vi "Define.vi"(11 "Collection Definition":T1) -> (3 "Entity Collection out":refnum<class "Entity Collection.lvclass">)   [LabVIEW 2020, in "Conditu2.lvlib" / "Columns.lvlib" / "Entity Collection.lvclass"]
uses:
  Entity Collection.lvclass
  C:/dev/lv20CE/lv-conditum-tools/Conditum-Clone/Columns/Relation/Relation.lvclass
  Collection Definition.ctl
  Relation/Relation Info.ctl
  Relation Mapping.ctl
  Relation/Relation Definition.ctl
  Type/Definition.ctl
  Type/Type.lvclass/Type.ctl
  Relation/Relation.lvclass/Relation.ctl
  Type/Define Type.vi
  Relation/Relation.lvclass
  C:/dev/lv20CE/lv-conditum-tools/Conditum-Clone/Columns/Type/Type.lvclass
  Type/Type.lvclass
  Conditu2.lvlib
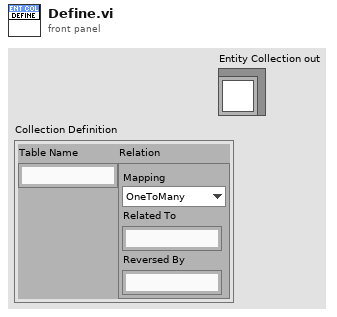
[diagram p1: front panel]
types:
  T1 = typedef "Conditu2.lvlib/Columns.lvlib/Entity Collection.lvclass/Collection Definition.ctl" = cluster{"Table Name":string, "Relation":T2}
  T2 = typedef "Conditu2.lvlib/Relation Info.ctl" = cluster{"Mapping":T3, "Related To":string, "Reversed By":string}
  T3 = typedef "Conditu2.lvlib/Relation Mapping.ctl" = enum16{"OneToMany", "ManyToOne", "ManyToMany", "OneToOne"}
  T4 = typedef "Conditu2.lvlib/Columns.lvlib/Relation.lvclass/Relation Definition.ctl" = cluster{"Type":T5, "Relation":T2}
  T5 = typedef "Conditu2.lvlib/Columns.lvlib/Type.lvclass/Definition.ctl" = cluster{"Name":string, "Nullable":bool, "Default NULL":bool}
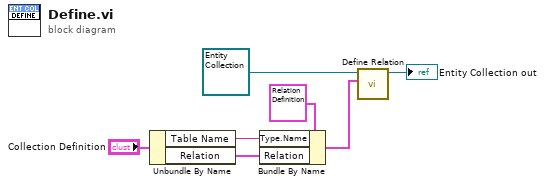
[diagram p0: block diagram]
diagram:
  n1 = Unbundle By Name("Collection Definition") -> ("Table Name"=w2:string, "Relation"=w1:T2)
  n2 = Bundle By Name(cluster=T4 {"Type"={"Name"="", "Nullable"=FALSE, "Default NULL"=FALSE}, "Relation"={"Mapping"=enum."OneToMany", "Related To"="", "Reversed By"=""}} ("Relation Definition"), "Type.Name"=w2, "Relation"=w1) -> (w3:T4)
  n3 = call "Define Relation.vi"("Relation Definition"=w3, "Relation in"=refnum<class "Entity Collection.lvclass"> refnum ("Entity Collection in")) -> ("Relation out"=→"Entity Collection out":refnum<class "Entity Collection.lvclass">)  [unwired: 9 in]
